vi "MeasureSinglePoint.vi"(7 "SMU":T1, 8 "Error In":errorcluster, 10 "Measure Function":T2, 11 "Keithley 2602 In":refnum<visa-resource-name>) -> (0 "Error Out":errorcluster, 2 "Reading":dbl, 3 "Keithley 2602 Out":refnum<visa-resource-name>)   [LabVIEW 2012, in "Keithley-2602.lvlib"]
uses:
  Keithley-2602.lvlib
  Controls/MeasureFunction.ctl
  Controls/SMU.ctl
panel:
  out "Command":string
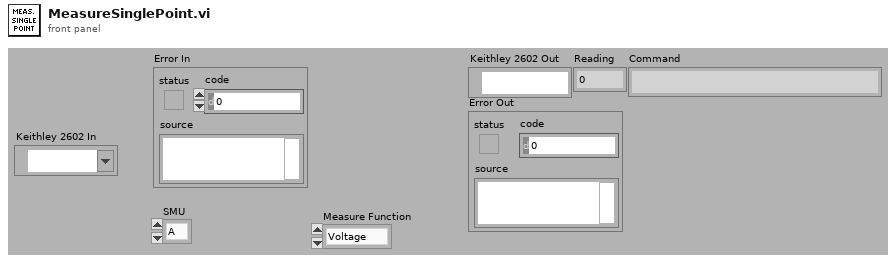
[diagram p1: front panel]
types:
  T1 = typedef "Keithley-2602.lvlib/SMU.ctl" = enum16{"A", "B"}
  T2 = typedef "Keithley-2602.lvlib/MeasureFunction.ctl" = enum16{"Voltage", "Current", "Resistance", "Power"}
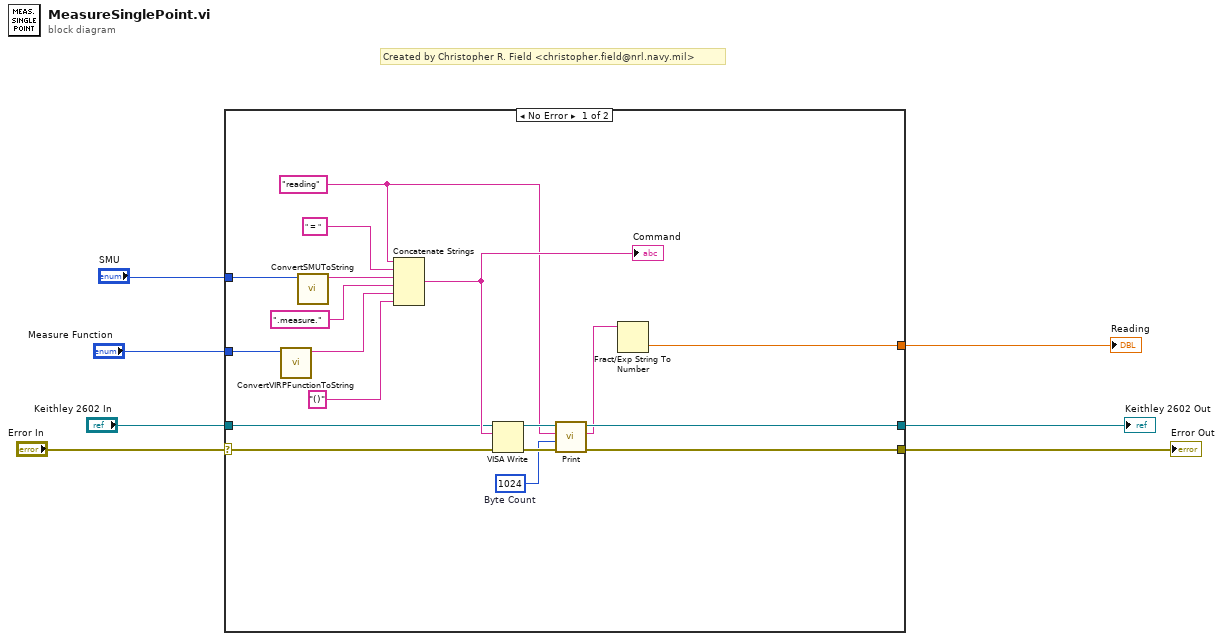
[diagram p0: block diagram]
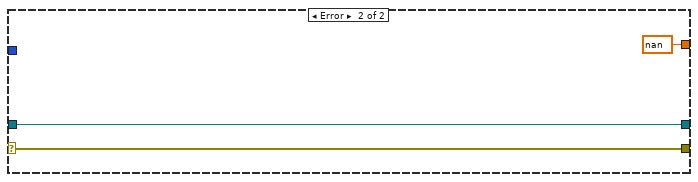
[diagram p2: hidden frame]
diagram:
  # "Created by Christopher R. Field <christopher.field@nrl.navy.mil>"
  n1 = case shown="No Error" "Error In" {
    selector: "Error In" -> [w9 w27]
    tunnel: "Keithley 2602 In" -> [w20 w28]
    tunnel: [w15 w28] -> w6
    tunnel: [w14 w27] -> w5
    tunnel: [w12 nan] -> w4
    tunnel: "SMU" -> [w11 _]
    tunnel: "Measure Function" -> [w10 _]
    frame No Error {
      w17 = u32 1024  # Byte Count
      w16 = "reading"
      n2 = call "ConvertVIRPFunctionToString.vi"("Function"=w10) -> ("Function"=w24:string)  [unwired: 10 in]
      n3 = call "ConvertSMUToString.vi"("SMU"=w11) -> ("Channel"=w25:string)  [unwired: 10 in]
      n4 = Concatenate Strings(w16, " = ", w25, ".measure.", w24, "()" ("string")) -> (w21:string)
      "Command" <- w21
      n5 = VISA Write(VISA resource name=w20, write buffer=w21, error in (no error)=w9) -> (VISA resource name out=w19:refnum<visa-resource-name>, error out=w18:errorcluster)  [unwired: 1 out]
      n6 = call "Print.vi"("Error In"=w18, "Byte Count"=w17, "Attribute"=w16, "Kiethley 2602 In"=w19) -> ("Error Out"=w14:errorcluster, "Output"=w13:string, "Keithley 2602 Out"=w15:refnum<visa-resource-name>)  [unwired: 5 in]
      n7 = Fract/Exp String To Number(string=w13) -> (number=w12:dbl)  [unwired: 3 in, 1 out]
    }
    frame Error {
    }
  }
  "Keithley 2602 Out" <- w6
  "Error Out" <- w5
  "Reading" <- w4
